vi "HFRR ADV v08.vi"() -> ()   [LabVIEW 2025] (continued)
                        "Humidity 2" <- w4456
                        n3193 = local write "Send"(w4457) -> ()
                        n3194 = local write "Ser Led"(w4457) -> ()
                        n3195 = VISA Read(VISA resource name=w4463, byte count=w4456, error in (no error)=w4464) -> (VISA resource name out=w4460:refnum<visa-resource-name>, read buffer=→"Humidity Str Rec":string, error out=w4459:errorcluster)  [unwired: 1 out]
                      }
                    }
                    n3196 = Select(t=w4434, s=w4435, f=w4432) -> (s? t:f=w4433:string)
                  }
                }
              }
              frame Error {
                w4480 = u16 0 items=["None"=0, "XON/XOFF"=1, "RTS/CTS"=2, "DTR/DSR"=4] ("flow control")
                w4476 = u16 0 items=["None", "Odd", "Even", "Mark", "Space"] ("parity")
                w4479 = u16 10 items=["1.0"=10, "1.5"=15, "2.0"=20] ("stop bits")
                n3197 = VISA Close(VISA resource name=w4472, error in (no error)=w4473) -> (error out=w4471:errorcluster)
                n3198 = local write "humid"("" ("humid")) -> ()
                n3199 = local write "Humidity Str Rec"("" ("Humidity Str Rec")) -> ()
                n3200 = call <vilib>:"Clear Errors.vi"("error in (no error)"=w4471) -> ("error out"=w4470:errorcluster)  [unwired: 5 in, 1 out]
                n3201 = local read "Com Port 3"() -> (w4469:refnum<visa-resource-name>)
                n3202 = call-poly "VISA Configure Serial Port"("VISA resource name"=w4469, "timeout (10sec)"=u32 1000, "termination char\n(0xA = '\\n' = LF)"=u8 10 ("termination char\n(0xA = '\\n' = LF)"), "Enable Termination\nChar (T)"=FALSE ("Enable Termination Char (T)"), "baud rate (9600)"="Humidity BaudRate", "data bits (8)"=u16 8 ("data bits"), "parity (0:none)"=w4476, "error in (no error)"=w4470, "stop bits (10: 1 bit)"=w4479, "flow control (0:none)"=w4480) -> ("VISA resource name out"=w4475:refnum<visa-resource-name>, "error out"=w4466:errorcluster)  [unwired: 4 in]
              }
            }
            n3203 = Compound Arithmetic op=AND(w4371, w4370, w4372) -> (w4369:bool)
            n3204 = case shown="True" w4369 {
              tunnel: w4368 -> [_ _]
              tunnel: w4377 -> [_ w4407]
              frame False {
              }
              frame True {
                w4405 = " " ("regular expression")
                n3205 = Match Pattern(string=w4407, regular expression=" ") -> (after substring=w4409:string)  [unwired: 1 in, 3 out]
                n3206 = Match Pattern(string=w4409, regular expression=w4405) -> (before substring=→"humid":string, after substring=w4406:string)  [unwired: 1 in, 2 out]
                n3207 = Match Pattern(string=w4406, regular expression=w4405) -> (before substring=→"temp_@Rh sensor":string)  [unwired: 1 in, 3 out]
              }
            }
            n3208 = local read "Quit"() -> (w4358:bool)
          }
          n3209 = VISA Close(VISA resource name=w4354, error in (no error)=w4355) -> (error out=w4351:errorcluster)
          n3210 = call <vilib>:"Clear Errors.vi"("error in (no error)"=w4351) -> ()  [unwired: 5 in, 2 out]
        }
        frame Enabled {
        }
      }
    }
    frame Enabled {
    }
  }
  n3211 = while {
    tunnel: [w4488] -> _
    i -> [w4488]
    stop <- w4483 stop-if-true
    # "Langauage selection"
    n3212 = property on="FF Calibration g" class="WFGraph (strict)"("Plot Area:Colors:FG Color"=u32 0) -> ()  [unwired: 2 in, 2 out]
    n3213 = Equal?(x="Lan flag", y=22.0) -> ()  [unwired: 1 out]
    n3214 = disable-structure shown="Disabled" {
      frame Disabled {
        n3215 = stacked-sequence {
          frame #0 {
            n3216 = case shown="\"Russian\"" "Language Selection" {
              tunnel: [0 1] -> w4490
              frame "English", Default {
              }
              frame "Russian" {
              }
            }
            n3217 = for {
              N: 130 -> [_]
              tunnel: "Table" -> [w4499]
              tunnel: w4490 -> [w4498]
              i -> [w4497]
              n3218 = Index Array(array=w4499, index (row)=w4497, index (col)=w4498) -> (element=w4496:string)
              n3219 = case shown="123" w4497 {
                tunnel: w4496 -> [w4500 w4501 _ w4502 w4503 w4504 w4505 w4506 w4507 w4508 w4509 w4510 w4511 w4512 w4513 w4514 w4515 w4516 w4517 w4518 w4519 w4520 w4521 w4522 w4523 w4524 w4525 w4526 w4527 _ _ w4528 w4529 w4530 w4531 w4532 w4533 w4542 w4549 w4556 w4563 w4567 w4570 w4573 w4575 w4577 w4578 w4579 w4580 w4581 w4582 w4583 w4584 w4585 w4586 w4587 w4588 w4589 w4590 w4591 w4592 w4593 w4594 w4595 w4596 w4597 w4598 w4599 w4600 w4601 w4602 w4603 w4604 w4605 w4606 w4607 w4608 w4609 w4610 w4611 w4612 w4613 w4614 w4615 w4616 w4617 w4618 w4619 w4620 w4621 w4622 w4623 w4624 w4625 w4626 w4627 w4628 w4629 w4630 w4631 w4632 w4633 w4634 w4635 w4636 _ w4637 w4638 w4639 w4640 w4641 w4642 w4643 w4644 w4645 w4646 w4647 w4648 w4649 _ w4650 w4651 w4652 w4653 w4654 w4655 _]
                frame 0 {
                  n3220 = local write "S"(w4500) -> ()
                }
                frame 1 {
                  n3221 = local write "S 2"(w4501) -> ()
                }
                frame 2 {
                }
                frame 3 {
                  n3222 = local write "S 4"(w4502) -> ()
                }
                frame 4 {
                  n3223 = property on="FILE" class="Str"("Caption.Text"=w4503) -> ()  [unwired: 2 in, 2 out]
                }
                frame 5 {
                  n3224 = property on="Fuel Discription :" class="Str"("Caption.Text"=w4504) -> ()  [unwired: 2 in, 2 out]
                }
                frame 6 {
                  n3225 = property on="Remarks :" class="Str"("Caption.Text"=w4505) -> ()  [unwired: 2 in, 2 out]
                }
                frame 7 {
                  n3226 = property on="Save & Continue" class="Bool (strict)"("Boolean Text.Text"=w4506) -> ()  [unwired: 2 in, 2 out]
                }
                frame 8 {
                }
                frame 9 {
                  n3227 = property on="Set Hz" class="DigNum (strict)"("Caption.Text"=w4508) -> ()  [unwired: 2 in, 2 out]
                }
                frame 10 {
                  "String 3" <- w4509
                }
                frame 11 {
                  n3228 = property on="NORMAL LOAD" class="DigNum (strict)"("Caption.Text"=w4510) -> ()  [unwired: 2 in, 2 out]
                }
                frame 12 {
                  "String 5" <- w4511
                }
                frame 13 {
                  n3229 = property on="Set Temp" class="DigNum (strict)"("Caption.Text"=w4512) -> ()  [unwired: 2 in, 2 out]
                }
                frame 14 {
                  n3230 = local write "S 15"(w4513) -> ()
                }
                frame 15 {
                  n3231 = property on="Set Rh" class="DigNum (strict)"("Caption.Text"=w4514) -> ()  [unwired: 2 in, 2 out]
                }
                frame 16 {
                  "String 13" <- w4515
                  "String 26" <- w4515
                }
                frame 17 {
                  n3232 = local write "S 18"(w4516) -> ()
                }
                frame 18 {
                  "String 17" <- w4517
                }
                frame 19 {
                  n3233 = property on="test time" class="DigNum (strict)"("Caption.Text"=w4518) -> ()  [unwired: 2 in, 2 out]
                }
                frame 20 {
                  "String 18" <- w4519
                  "String 22" <- w4519
                }
                frame 21 {
                  n3234 = property on="Elapsed time" class="DigNum (strict)"("Caption.Text"=w4520) -> ()  [unwired: 2 in, 2 out]
                }
                frame 22 {
                  n3235 = property on="Samplingtime 2" class="DigNum (strict)"("Caption.Text"=w4521) -> ()  [unwired: 2 in, 2 out]
                }
                frame 23 {
                  "String 21" <- w4522
                }
                frame 24 {
                  n3236 = property on="Countdown" class="DigNum (strict)"("Caption.Text"=w4523) -> ()  [unwired: 2 in, 2 out]
                }
                frame 25 {
                  n3237 = property on="Countdown 2" class="DigNum (strict)"("Caption.Text"=w4524) -> ()  [unwired: 2 in, 2 out]
                }
                frame 26 {
                  n3238 = property on="Engage" class="Bool (strict)"("Boolean Text.Text"=w4525) -> ()  [unwired: 2 in, 2 out]
                }
                frame 27 {
                  n3239 = property on="Boolean  4" class="Bool (strict)"("Boolean Text.Text"=w4526) -> ()  [unwired: 2 in, 2 out]
                }
                frame 28 {
                  n3240 = property on="Test \nStatus" class="Bool (strict)"("Boolean Text.Text"=w4527) -> ()  [unwired: 2 in, 2 out]
                }
                frame 29 {
                }
                frame 30 {
                }
                frame 31 {
                  n3241 = property on="FF Calibration g" class="WFGraph (strict)"("X Scale.Name Label.Text"=w4528) -> ()  [unwired: 2 in, 2 out]
                }
                frame 32 {
                  n3242 = property on="RSTCOF" class="Bool"("Boolean Text.Text"=w4529) -> ()  [unwired: 2 in, 2 out]
                  n3243 = property on="RST FF" class="Bool"("Boolean Text.Text"=w4529) -> ()  [unwired: 2 in, 2 out]
                  n3244 = property on="RST TEMP" class="Bool"("Boolean Text.Text"=w4529) -> ()  [unwired: 2 in, 2 out]
                  n3245 = property on="RSTV1 3" class="Bool"("Boolean Text.Text"=w4529) -> ()  [unwired: 2 in, 2 out]
                  n3246 = property on="rstv2" class="Bool"("Boolean Text.Text"=w4529) -> ()  [unwired: 2 in, 2 out]
                  n3247 = property on="RSTV1 2" class="Bool"("Boolean Text.Text"=w4529) -> ()  [unwired: 2 in, 2 out]
                  n3248 = property on="RST CP" class="Bool"("Boolean Text.Text"=w4529) -> ()  [unwired: 2 in, 2 out]
                }
                frame 33 {
                  "S 61" <- w4530
                }
                frame 34 {
                  "String 23" <- w4531
                }
                frame 35 {
                  n3249 = property on="Rh Before" class="DigNum (strict)"("Caption.Text"=w4532) -> ()  [unwired: 2 in, 2 out]
                }
                frame 36 {
                  n3250 = Match Pattern(string=w4533, regular expression=",") -> (before substring=→"bs":string, after substring=→"as":string)  [unwired: 1 in, 2 out]
                  n3251 = property on="Rh After" class="DigNum (strict)"("Caption.Text"=w4533) -> ()  [unwired: 2 in, 2 out]
                }
                frame 37 {
                  n3252 = Match Pattern(string=w4542, regular expression=",") -> (before substring=w4541:string, after substring=w4540:string)  [unwired: 1 in, 2 out]
                  "bs" <- w4541
                  "as" <- w4540
                  n3253 = Concatenate Strings(w4541, w4540) -> (w4537:string)
                  n3254 = property on="Humidity before test 2" class="DigNum (strict)"("Caption.Text"=w4537) -> ()  [unwired: 2 in, 2 out]
                  n3255 = property on="Humidity before test" class="DigNum (strict)"("Caption.Text"=w4537) -> ()  [unwired: 2 in, 2 out]
                  n3256 = Concatenate Strings(w4537, "=" ("string")) -> (w4538:string)
                  n3257 = local write "S 38"(w4538) -> ()
                }
                frame 38 {
                  n3258 = Match Pattern(string=w4549, regular expression=",") -> (before substring=w4548:string, after substring=w4547:string)  [unwired: 1 in, 2 out]
                  "bs" <- w4548
                  "as" <- w4547
                  n3259 = Concatenate Strings(w4548, w4547) -> (w4544:string)
                  n3260 = property on="Humidity after test 2" class="DigNum (strict)"("Caption.Text"=w4544) -> ()  [unwired: 2 in, 2 out]
                  n3261 = Concatenate Strings(w4544, "=" ("string")) -> (w4546:string)
                  n3262 = property on="Humidity after test" class="DigNum (strict)"("Caption.Text"=w4544) -> ()  [unwired: 2 in, 2 out]
                  n3263 = local write "S 39"(w4546) -> ()
                }
                frame 39 {
                  n3264 = Match Pattern(string=w4556, regular expression=",") -> (before substring=w4555:string, after substring=w4554:string)  [unwired: 1 in, 2 out]
                  "bs" <- w4555
                  "as" <- w4554
                  n3265 = Concatenate Strings(w4555, w4554) -> (w4551:string)
                  n3266 = property on="Temperature before test 2" class="DigNum (strict)"("Caption.Text"=w4551) -> ()  [unwired: 2 in, 2 out]
                  n3267 = property on="Temperature before test" class="DigNum (strict)"("Caption.Text"=w4551) -> ()  [unwired: 2 in, 2 out]
                  n3268 = Concatenate Strings(w4551, "=" ("string")) -> (→"String 34":string)
                }
                frame 40 {
                  n3269 = Match Pattern(string=w4563, regular expression=",") -> (before substring=w4562:string, after substring=w4561:string)  [unwired: 1 in, 2 out]
                  "bs" <- w4562
                  "as" <- w4561
                  n3270 = Concatenate Strings(w4562, w4561) -> (w4558:string)
                  n3271 = property on="Temperature after test 2" class="DigNum (strict)"("Caption.Text"=w4558) -> ()  [unwired: 2 in, 2 out]
                  n3272 = Concatenate Strings(w4558, "=" ("string")) -> (→"String 35":string)
                  n3273 = property on="Temperature after test" class="DigNum (strict)"("Caption.Text"=w4558) -> ()  [unwired: 2 in, 2 out]
                }
                frame 41 {
                  n3274 = property on="AVP" class="DigNum (strict)"("Caption.Text"=w4567) -> ()  [unwired: 2 in, 2 out]
                  n3275 = property on="AVP 2" class="DigNum (strict)"("Caption.Text"=w4567) -> ()  [unwired: 2 in, 2 out]
                  n3276 = Concatenate Strings(w4567, "=" ("string")) -> (→"String 36":string)
                }
                frame 42 {
                  n3277 = property on="MWSD" class="DigNum (strict)"("Caption.Text"=w4570) -> ()  [unwired: 2 in, 2 out]
                  n3278 = property on="MWSD 2" class="DigNum (strict)"("Caption.Text"=w4570) -> ()  [unwired: 2 in, 2 out]
                  n3279 = Concatenate Strings(w4570, "=" ("string")) -> (→"String 37":string)
                }
                frame 43 {
                  n3280 = property on="HCF 2" class="DigNum (strict)"("Caption.Text"=w4573) -> ()  [unwired: 2 in, 2 out]
                  n3281 = property on="HCF" class="DigNum (strict)"("Caption.Text"=w4573) -> ()  [unwired: 2 in, 2 out]
                  n3282 = Concatenate Strings(w4573, "=" ("string")) -> (→"String 38":string)
                }
                frame 44 {
                  n3283 = Concatenate Strings(w4575, "=" ("string")) -> (→"String 39":string)
                  n3284 = property on="WS1.4 2" class="DigNum (strict)"("Caption.Text"=w4575) -> ()  [unwired: 2 in, 2 out]
                  n3285 = property on="WS1.4" class="DigNum (strict)"("Caption.Text"=w4575) -> ()  [unwired: 2 in, 2 out]
                }
                frame 45 {
                  n3286 = property on="Save Results" class="Bool (strict)"("Boolean Text.Text"=w4577) -> ()  [unwired: 2 in, 2 out]
                }
                frame 46 {
                  n3287 = local write "S 47"(w4578) -> ()
                }
                frame 47 {
                  n3288 = local write "S 48"(w4579) -> ()
                }
                frame 48 {
                  n3289 = local write "S 49"(w4580) -> ()
                }
                frame 49 {
                  n3290 = local write "S 50"(w4581) -> ()
                }
                frame 50 {
                  n3291 = local write "S 51"(w4582) -> ()
                }
                frame 51 {
                  n3292 = local write "S 52"(w4583) -> ()
                }
                frame 52 {
                  n3293 = local write "S 53"(w4584) -> ()
                }
                frame 53 {
                  n3294 = local write "S 54"(w4585) -> ()
                }
                frame 54 {
                  n3295 = local write "S 55"(w4586) -> ()
                }
                frame 55 {
                  n3296 = local write "S 56"(w4587) -> ()
                }
                frame 56 {
                  n3297 = local write "S 57"(w4588) -> ()
                }
                frame 57 {
                  n3298 = local write "S 58"(w4589) -> ()
                }
                frame 58 {
                  n3299 = local write "S 59"(w4590) -> ()
                }
                frame 59 {
                  n3300 = local write "S 60"(w4591) -> ()
                }
                frame 60 {
                  n3301 = local write "S 62"(w4592) -> ()
                }
                frame 61 {
                  n3302 = local write "S 63"(w4593) -> ()
                }
                frame 62 {
                  n3303 = local write "S 64"(w4594) -> ()
                }
                frame 63 {
                  n3304 = local write "S 65"(w4595) -> ()
                }
                frame 64 {
                  n3305 = local write "S 66"(w4596) -> ()
                }
                frame 65 {
                  n3306 = local write "S 67"(w4597) -> ()
                }
                frame 66 {
                  n3307 = local write "S 68"(w4598) -> ()
                }
                frame 67 {
                  n3308 = local write "S 69"(w4599) -> ()
                }
                frame 68 {
                  n3309 = local write "S 70"(w4600) -> ()
                }
                frame 69 {
                  n3310 = local write "S 71"(w4601) -> ()
                }
                frame 70 {
                  n3311 = local write "S 72"(w4602) -> ()
                }
                frame 71 {
                  n3312 = local write "S 73"(w4603) -> ()
                }
                frame 72 {
                  n3313 = local write "S 74"(w4604) -> ()
                }
                frame 73 {
                  n3314 = local write "S 75"(w4605) -> ()
                }
                frame 74 {
                  n3315 = local write "S 76"(w4606) -> ()
                }
                frame 75 {
                  n3316 = local write "S 77"(w4607) -> ()
                }
                frame 76 {
                  n3317 = local write "S 78"(w4608) -> ()
                }
                frame 77 {
                  n3318 = local write "S 79"(w4609) -> ()
                }
                frame 79 {
                  n3319 = property on="Sample Temperature ( °C )" class="XYGraph (strict)"("Y Scale.Name Label.Text"=w4610) -> ()  [unwired: 2 in, 2 out]
                }
                frame 80 {
                  n3320 = local write "S 81"(w4611) -> ()
                  n3321 = property on="Humidity ( %RH )" class="XYGraph (strict)"("Y Scale.Name Label.Text"=w4611) -> ()  [unwired: 2 in, 2 out]
                }
                frame 78 {
                  n3322 = property on="Air Temperature  ( °C )" class="XYGraph (strict)"("X Scale.Name Label.Text"=w4612) -> ()  [unwired: 2 in, 2 out]
                  n3323 = property on="Humidity ( %RH )" class="XYGraph (strict)"("X Scale.Name Label.Text"=w4612) -> ()  [unwired: 2 in, 2 out]
                  n3324 = property on="Sample Temperature ( °C )" class="XYGraph (strict)"("X Scale.Name Label.Text"=w4612) -> ()  [unwired: 2 in, 2 out]
                  n3325 = property on="Coefficient Of Friction" class="XYGraph (strict)"("X Scale.Name Label.Text"=w4612) -> ()  [unwired: 2 in, 2 out]
                }
                frame 81 {
                  n3326 = property on="Air Temperature  ( °C )" class="XYGraph (strict)"("Y Scale.Name Label.Text"=w4613) -> ()  [unwired: 2 in, 2 out]
                }
                frame 82 {
                  n3327 = local write "S 84"(w4614) -> ()
                }
                frame 83 {
                  n3328 = local write "S 85"(w4615) -> ()
                }
                frame 84 {
                  n3329 = local write "S 86"(w4616) -> ()
                }
                frame 85 {
                  n3330 = local write "S 87"(w4617) -> ()
                }
                frame 86 {
                  n3331 = local write "S 88"(w4618) -> ()
                }
                frame 87 {
                  n3332 = property on="FF Calibration g" class="WFGraph (strict)"("Y Scale.Name Label.Text"=w4619) -> ()  [unwired: 2 in, 2 out]
                }
                frame 88 {
                  n3333 = local write "S 90"(w4620) -> ()
                }
                frame 89 {
                  n3334 = local write "S 91"(w4621) -> ()
                }
                frame 90 {
                  n3335 = local write "S 92"(w4622) -> ()
                }
                frame 91 {
                  n3336 = local write "S 93"(w4623) -> ()
                }
                frame 92 {
                  n3337 = local write "S 94"(w4624) -> ()
                }
                frame 93 {
                  n3338 = local write "S 95"(w4625) -> ()
                }
                frame 94 {
                  n3339 = local write "S 96"(w4626) -> ()
                }
                frame 95 {
                  n3340 = local write "S 97"(w4627) -> ()
                }
                frame 96 {
                  n3341 = local write "S 98"(w4628) -> ()
                }
                frame 97 {
                  n3342 = local write "S 99"(w4629) -> ()
                }
                frame 98 {
                  n3343 = local write "S 100"(w4630) -> ()
                }
                frame 99 {
                  n3344 = local write "S 101"(w4631) -> ()
                }
                frame 100 {
                  n3345 = local write "S 102"(w4632) -> ()
                }
                frame 101 {
                  n3346 = local write "S 103"(w4633) -> ()
                }
                frame 102 {
                  n3347 = local write "S 104"(w4634) -> ()
                }
                frame 103 {
                  n3348 = local write "S 105"(w4635) -> ()
                }
                frame 104 {
                  n3349 = local write "S 106"(w4636) -> ()
                }
                frame 105 {
                }
                frame 106 {
                  n3350 = property on="OK Button 17" class="Bool (strict)"("Boolean Text.Text"=w4637) -> ()  [unwired: 2 in, 2 out]
                }
                frame 107 {
                  n3351 = property on="OK Button 16" class="Bool (strict)"("Boolean Text.Text"=w4638) -> ()  [unwired: 2 in, 2 out]
                }
                frame 108 {
                  n3352 = property on="TITTLE" class="Str"("Caption.Text"=w4639) -> ()  [unwired: 2 in, 2 out]
                }
                frame 109 {
                  "String 30" <- w4640
                }
                frame 110 {
                  n3353 = property on="Test Date" class="Str"("Caption.Text"=w4641) -> ()  [unwired: 2 in, 2 out]
                  "String 31" <- w4641
                }
                frame 111 {
                  n3354 = property on="Sample ID" class="Str"("Caption.Text"=w4642) -> ()  [unwired: 2 in, 2 out]
                  "String 32" <- w4642
                }
                frame 112 {
                  n3355 = property on="Tested by" class="Str"("Caption.Text"=w4643) -> ()  [unwired: 2 in, 2 out]
                  "String 33" <- w4643
                }
                frame 113 {
                  n3356 = property on="System Configured Printers 2" class="Arr (strict)"("Caption.Text"=w4644) -> ()  [unwired: 2 in, 2 out]
                }
                frame 114 {
                  n3357 = property on="Selected Printer" class="Str"("Caption.Text"=w4645) -> ()  [unwired: 2 in, 2 out]
                }
                frame 115 {
                  n3358 = property on="Select Printer 3" class="DigNum (strict)"("Caption.Text"=w4646) -> ()  [unwired: 2 in, 2 out]
                }
                frame 116 {
                  n3359 = property on="Print" class="Bool (strict)"("Boolean Text.Text"=w4647) -> ()  [unwired: 2 in, 2 out]
                }
                frame 117 {
                  "String 41" <- w4648
                }
                frame 118 {
                  n3360 = property on="tested by" class="Str"("Caption.Text"=w4649) -> ()  [unwired: 2 in, 2 out]
                }
                frame 119 {
                }
                frame 120 {
                  n3361 = property on="Export" class="Bool (strict)"("Boolean Text.Text"=w4650) -> ()  [unwired: 2 in, 2 out]
                }
                frame 121 {
                  n3362 = property on="TEMP INTERCEPT:" class="DigNum (strict)"("Caption.Text"=w4651) -> ()  [unwired: 2 in, 2 out]
                }
                frame 122 {
                  n3363 = property on="AIR TEMP INTERCEPT:" class="DigNum (strict)"("Caption.Text"=w4652) -> ()  [unwired: 2 in, 2 out]
                }
                frame 123 {
                  n3364 = property on="Select File Type" class="Enum (strict)"("Caption.Text"=w4653) -> ()  [unwired: 2 in, 2 out]
                }
                frame 124 {
                  n3365 = property on="s.NO" class="Str"("Caption.Text"=w4654) -> ()  [unwired: 2 in, 2 out]
                  "String 45" <- w4654
                }
                frame 125 {
                  n3366 = property on="trip1 8" class="Bool (strict)"("Boolean Text.Text"=w4655) -> ()  [unwired: 2 in, 2 out]
                }
                frame 126, Default {
                }
              }
            }
          }
          frame #1 {
            w4663 = TRUE ("Visible")
            n3367 = local read "S 91"() -> (w4680:string)
            n3368 = local read "S 90"() -> (w4679:string)
            n3369 = local read "S 88"() -> (w4678:string)
            n3370 = property on="Threshold" class="DigNum (strict)"("Caption.Text"=w4680) -> ()  [unwired: 2 in, 2 out]
            n3371 = property on="File Path" class="Path"("Caption.Text"=w4679) -> ()  [unwired: 2 in, 2 out]
            n3372 = property on="SrvM CP" class="Bool (strict)"("Boolean Text.Text"=w4678) -> ()  [unwired: 2 in, 2 out]
            n3373 = local read "S 71"() -> (w4673:string)
            n3374 = local read "S 86"() -> (w4675:string)
            n3375 = local read "S 85"() -> (w4676:string)
            n3376 = local read "S 87"() -> (w4674:string)
            n3377 = local read "S 84"() -> (w4677:string)
            n3378 = local read "S 103"() -> (w4662:string)
            n3379 = local read "S 104"() -> (w4661:string)
            n3380 = property on="ENTER THE NEW PASSWORD" class="Str"("Caption.Text"=w4674) -> ()  [unwired: 2 in, 2 out]
            n3381 = property on="Password" class="Str"("Caption.Text"=w4676) -> ()  [unwired: 2 in, 2 out]
            n3382 = property on="ENTER CURRENT PASSWORD" class="Str"("Caption.Text"=w4675) -> ()  [unwired: 2 in, 2 out]
            n3383 = property on="EDIT" class="Bool (strict)"("Boolean Text.Text"=w4673) -> ()  [unwired: 2 in, 2 out]
            n3384 = property on="SAVE" class="Bool (strict)"("Boolean Text.Text"=w4677) -> ()  [unwired: 2 in, 2 out]
            n3385 = Build Array(w4662, w4661) -> (w4660:string[])
            n3386 = property on="Heater Button" class="Bool (strict)"("Strings [4]"=w4660) -> ()  [unwired: 2 in, 2 out]
            n3387 = property on="CH-HUMIDITY WET" class="DigNum (strict)"("Caption.Size to Text?"=w4663) -> ()  [unwired: 2 in, 2 out]
            n3388 = property on="CH-HUMIDITY DRY" class="DigNum (strict)"("Caption.Size to Text?"=w4663) -> ()  [unwired: 2 in, 2 out]
            n3389 = property on="CH-POWER -" class="DigNum (strict)"("Caption.Size to Text?"=w4663) -> ()  [unwired: 2 in, 2 out]
            n3390 = property on="CH-HEATER" class="DigNum (strict)"("Caption.Size to Text?"=w4663) -> ()  [unwired: 2 in, 2 out]
            n3391 = property on="CH-POWER +" class="DigNum (strict)"("Caption.Size to Text?"=w4663) -> ()  [unwired: 2 in, 2 out]
            n3392 = local read "S 92"() -> (w4672:string)
            n3393 = local read "S 93"() -> (w4671:string)
            n3394 = local read "S 105"() -> (w4658:string)
            n3395 = local read "S 106"() -> (w4657:string)
            n3396 = Build Array(w4672, w4671) -> ()  [unwired: 1 out]
            n3397 = Build Array(w4658, w4657) -> (w4659:string[])
            n3398 = local read "S 95"() -> (w4669:string)
            n3399 = local read "S 94"() -> (w4670:string)
            n3400 = local read "bs"() -> (w4685:string)
            n3401 = local read "as"() -> (w4686:string)
            n3402 = property on="Humidity" class="Bool (strict)"("Strings [4]"=w4659) -> ()  [unwired: 2 in, 2 out]
            n3403 = Concatenate Strings(w4685, "\r", w4686) -> ()  [unwired: 1 out]
            n3404 = property on="STROKE GAIN :" class="DigNum (strict)"("Caption.Text"=w4669) -> ()  [unwired: 2 in, 2 out]
            n3405 = property on="DISPLACEMENT :" class="DigNum (strict)"("Caption.Text"=w4670) -> ()  [unwired: 2 in, 2 out]
            n3406 = property on="Rh After" class="DigNum (strict)"("Caption.Size to Text?"=TRUE ("Caption.Size to Text")) -> ()  [unwired: 2 in, 2 out]
            n3407 = local read "S 48"() -> (w4709:string)
            n3408 = local read "S 50"() -> (w4707:string)
            n3409 = local read "S 51"() -> (w4706:string)
            n3410 = local read "S 49"() -> (w4708:string)
            n3411 = local read "S 52"() -> (w4705:string)
            n3412 = local read "as"() -> (w4690:string)
            n3413 = local read "bs"() -> (w4691:string)
            n3414 = local read "S 56"() -> (w4704:string)
            n3415 = local read "S 57"() -> (w4703:string)
            n3416 = local read "S 58"() -> (w4702:string)
            n3417 = local read "S 59"() -> (w4701:string)
            n3418 = property on="OPEN" class="Bool (strict)"("Boolean Text.Text"=w4705) -> ()  [unwired: 2 in, 2 out]
            n3419 = property on="OPEN 1" class="Bool (strict)"("Boolean Text.Text"=w4709) -> ()  [unwired: 2 in, 2 out]
            n3420 = property on="OPEN 2" class="Bool (strict)"("Boolean Text.Text"=w4708) -> ()  [unwired: 2 in, 2 out]
            n3421 = property on="OPEN 3" class="Bool (strict)"("Boolean Text.Text"=w4707) -> ()  [unwired: 2 in, 2 out]
            n3422 = property on="OPEN 4" class="Bool (strict)"("Boolean Text.Text"=w4706) -> ()  [unwired: 2 in, 2 out]
            n3423 = Concatenate Strings(w4691, "\r", w4690) -> ()  [unwired: 1 out]
            n3424 = local read "S 102"() -> (w4664:string)
            n3425 = property on="КОФ1" class="DigNum (strict)"("Caption.Text"=w4704) -> ()  [unwired: 2 in, 2 out]
            n3426 = local read "S 98"() -> (w4668:string)
            n3427 = local read "S 99"() -> (w4667:string)
            n3428 = local read "S 100"() -> (w4666:string)
            n3429 = local read "S 101"() -> (w4665:string)
            n3430 = property on="КОФ2" class="DigNum (strict)"("Caption.Text"=w4703) -> ()  [unwired: 2 in, 2 out]
            n3431 = property on="КОФ3" class="DigNum (strict)"("Caption.Text"=w4702) -> ()  [unwired: 2 in, 2 out]
            n3432 = property on="КОФ4" class="DigNum (strict)"("Caption.Text"=w4701) -> ()  [unwired: 2 in, 2 out]
            n3433 = local read "bs"() -> (w4689:string)
            n3434 = local read "as"() -> (w4688:string)
            n3435 = property on="CH-POWER +" class="DigNum (strict)"("Caption.Text"=w4668) -> ()  [unwired: 2 in, 2 out]
            n3436 = property on="CH-POWER -" class="DigNum (strict)"("Caption.Text"=w4667) -> ()  [unwired: 2 in, 2 out]
            n3437 = property on="CH-HEATER" class="DigNum (strict)"("Caption.Text"=w4666) -> ()  [unwired: 2 in, 2 out]
            n3438 = property on="CH-HUMIDITY DRY" class="DigNum (strict)"("Caption.Text"=w4665) -> ()  [unwired: 2 in, 2 out]
            n3439 = property on="CH-HUMIDITY WET" class="DigNum (strict)"("Caption.Text"=w4664) -> ()  [unwired: 2 in, 2 out]
            n3440 = local read "S 60"() -> (w4700:string)
            n3441 = local read "S 54"() -> (w4710:string)
            n3442 = Concatenate Strings(w4689, "\r", w4688) -> ()  [unwired: 1 out]
            n3443 = Concatenate Strings(w4710, w4700) -> ()  [unwired: 1 out]
            n3444 = local read "S 77"() -> (→"String 43":string)
            n3445 = local read "S 76"() -> (w4683:string)
            n3446 = local read "S 78"() -> (w4682:string)
            n3447 = local read "S 71"() -> (w4694:string)
            n3448 = local read "S 66"() -> (w4699:string)
            n3449 = local read "S 67"() -> (w4698:string)
            n3450 = local read "S 68"() -> (w4697:string)
            n3451 = local read "S 69"() -> (w4696:string)
            n3452 = local read "S 70"() -> (w4695:string)
            n3453 = property on="AIR TEMP" class="DigNum (strict)"("Caption.Text"=w4682) -> ()  [unwired: 2 in, 2 out]
            n3454 = property on="Set Strk" class="DigNum (strict)"("Caption.Text"=w4683) -> ()  [unwired: 2 in, 2 out]
            n3455 = property on="FRIC. FORCE :" class="DigNum (strict)"("Caption.Text"=w4699) -> ()  [unwired: 2 in, 2 out]
            n3456 = property on="TEMPERATURE :" class="DigNum (strict)"("Caption.Text"=w4698) -> ()  [unwired: 2 in, 2 out]
            n3457 = property on="SPEED OUT:" class="DigNum (strict)"("Caption.Text"=w4697) -> ()  [unwired: 2 in, 2 out]
            n3458 = property on="AIR TEMPERATURE :" class="DigNum (strict)"("Caption.Text"=w4696) -> ()  [unwired: 2 in, 2 out]
            n3459 = property on="HUMIDITY:" class="DigNum (strict)"("Caption.Text"=w4695) -> ()  [unwired: 2 in, 2 out]
            n3460 = property on="EDIT" class="Bool (strict)"("Boolean Text.Text"=w4694) -> ()  [unwired: 2 in, 2 out]
            n3461 = local read "S 79"() -> (w4681:string)
            n3462 = property on="Stroke" class="DigNum (strict)"("Caption.Text"=w4681) -> ()  [unwired: 2 in, 2 out]
          }
          frame #2 {
          }
        }
        n3463 = local write "Lan flag"(10.0 ("Lan flag")) -> ()
      }
      frame Enabled {
      }
    }
    n3464 = Wait (ms)(milliseconds to wait=u32 2000) -> ()  [unwired: 1 out]
    n3465 = local read "Quit"() -> (w4483:bool)
  }
  n3466 = disable-structure shown="Disabled" {
    frame Disabled {
      n3467 = while {
        tunnel: [w4712] -> _
        i -> [w4712]
        stop <- w4711 continue-if-true
        n3468 = Wait (ms)(milliseconds to wait=u32 50) -> ()  [unwired: 1 out]
        n3469 = stacked-sequence {
          frame #0 {
            # "Controls Text color"
            # "Controls BG color"
            n3470 = property on="FILE" class="Str"("Text.Text Colors:Text Color"="SC  Text") -> ()  [unwired: 2 in, 2 out]
            n3471 = property on="Fuel Discription :" class="Str"("Text.Text Colors:Text Color"="SC  Text") -> ()  [unwired: 2 in, 2 out]
            n3472 = property on="tested by" class="Str"("Text.Text Colors:Text Color"="SC  Text") -> ()  [unwired: 2 in, 2 out]
            n3473 = property on="Remarks :" class="Str"("Text.Text Colors:Text Color"="SC  Text") -> ()  [unwired: 2 in, 2 out]
            n3474 = property class="DigNum (strict)"("Numeric Text.Text Colors:BG Color"="NC BG") -> ()  [unwired: 2 in, 2 out]
            n3475 = property class="DigNum (strict)"("Numeric Text.Text Colors:BG Color"="NC BG") -> ()  [unwired: 2 in, 2 out]
            n3476 = property class="DigNum (strict)"("Numeric Text.Text Colors:BG Color"="NC BG") -> ()  [unwired: 2 in, 2 out]
            n3477 = property class="DigNum (strict)"("Numeric Text.Text Colors:BG Color"="NC BG") -> ()  [unwired: 2 in, 2 out]
            n3478 = property class="DigNum (strict)"("Numeric Text.Text Colors:BG Color"="NC BG") -> ()  [unwired: 2 in, 2 out]
            n3479 = property class="DigNum (strict)"("Numeric Text.Text Colors:BG Color"="NC BG") -> ()  [unwired: 2 in, 2 out]
            n3480 = property class="DigNum (strict)"("Numeric Text.Text Colors:BG Color"="NC BG") -> ()  [unwired: 2 in, 2 out]
            n3481 = property class="DigNum (strict)"("Numeric Text.Text Colors:BG Color"="NC BG") -> ()  [unwired: 2 in, 2 out]
            n3482 = property class="DigNum (strict)"("Numeric Text.Text Colors:BG Color"="NC BG") -> ()  [unwired: 2 in, 2 out]
            n3483 = property class="DigNum (strict)"("Numeric Text.Text Colors:BG Color"="NC BG") -> ()  [unwired: 2 in, 2 out]
            n3484 = property class="DigNum (strict)"("Numeric Text.Text Colors:BG Color"="NC BG") -> ()  [unwired: 2 in, 2 out]
            n3485 = property class="DigNum (strict)"("Numeric Text.Text Colors:BG Color"="NC BG") -> ()  [unwired: 2 in, 2 out]
            n3486 = property on="FILE" class="Str"("Text.Text Colors:BG Color"="SC BG 3") -> ()  [unwired: 2 in, 2 out]
            n3487 = property on="Fuel Discription :" class="Str"("Text.Text Colors:BG Color"="SC BG 3") -> ()  [unwired: 2 in, 2 out]
            n3488 = property on="tested by" class="Str"("Text.Text Colors:BG Color"="SC BG 3") -> ()  [unwired: 2 in, 2 out]
            n3489 = property on="Remarks :" class="Str"("Text.Text Colors:BG Color"="SC BG 3") -> ()  [unwired: 2 in, 2 out]
            n3490 = property class="DigNum (strict)"("Numeric Text.Text Colors:Text Color"="NC Text") -> ()  [unwired: 2 in, 2 out]
            n3491 = property class="DigNum (strict)"("Numeric Text.Text Colors:Text Color"="NC Text") -> ()  [unwired: 2 in, 2 out]
            n3492 = property class="DigNum (strict)"("Numeric Text.Text Colors:Text Color"="NC Text") -> ()  [unwired: 2 in, 2 out]
            n3493 = property class="DigNum (strict)"("Numeric Text.Text Colors:Text Color"="NC Text") -> ()  [unwired: 2 in, 2 out]
            n3494 = property class="DigNum (strict)"("Numeric Text.Text Colors:Text Color"="NC Text") -> ()  [unwired: 2 in, 2 out]
            n3495 = property class="DigNum (strict)"("Numeric Text.Text Colors:Text Color"="NC Text") -> ()  [unwired: 2 in, 2 out]
            n3496 = property class="DigNum (strict)"("Numeric Text.Text Colors:Text Color"="NC Text") -> ()  [unwired: 2 in, 2 out]
            n3497 = property class="DigNum (strict)"("Numeric Text.Text Colors:Text Color"="NC Text") -> ()  [unwired: 2 in, 2 out]
            n3498 = property class="DigNum (strict)"("Numeric Text.Text Colors:Text Color"="NC Text") -> ()  [unwired: 2 in, 2 out]
            n3499 = property class="DigNum (strict)"("Numeric Text.Text Colors:Text Color"="NC Text") -> ()  [unwired: 2 in, 2 out]
            n3500 = property class="DigNum (strict)"("Numeric Text.Text Colors:Text Color"="NC Text") -> ()  [unwired: 2 in, 2 out]
            n3501 = property class="DigNum (strict)"("Numeric Text.Text Colors:Text Color"="NC Text") -> ()  [unwired: 2 in, 2 out]
            n3502 = property class="DigNum (strict)"("Numeric Text.Text Colors:Text Color"="NI Text  2") -> ()  [unwired: 2 in, 2 out]
            n3503 = property class="DigNum (strict)"("Numeric Text.Text Colors:Text Color"="NI Text  2") -> ()  [unwired: 2 in, 2 out]
            n3504 = property class="DigNum (strict)"("Numeric Text.Text Colors:Text Color"="NI Text  2") -> ()  [unwired: 2 in, 2 out]
            n3505 = property class="DigNum (strict)"("Numeric Text.Text Colors:Text Color"="NI Text  2") -> ()  [unwired: 2 in, 2 out]
            n3506 = property class="DigNum (strict)"("Numeric Text.Text Colors:Text Color"="NI Text  2") -> ()  [unwired: 2 in, 2 out]
            n3507 = property class="DigNum (strict)"("Numeric Text.Text Colors:Text Color"="NI Text  2") -> ()  [unwired: 2 in, 2 out]
            n3508 = property class="DigNum (strict)"("Numeric Text.Text Colors:Text Color"="NI Text  2") -> ()  [unwired: 2 in, 2 out]
            n3509 = property class="DigNum (strict)"("Numeric Text.Text Colors:Text Color"="NI Text  2") -> ()  [unwired: 2 in, 2 out]
            n3510 = property class="DigNum (strict)"("Numeric Text.Text Colors:Text Color"="NI Text  2") -> ()  [unwired: 2 in, 2 out]
            n3511 = property class="DigNum (strict)"("Numeric Text.Text Colors:Text Color"="NI Text  2") -> ()  [unwired: 2 in, 2 out]
            n3512 = property class="DigNum (strict)"("Numeric Text.Text Colors:Text Color"="NI Text  2") -> ()  [unwired: 2 in, 2 out]
            n3513 = property class="DigNum (strict)"("Numeric Text.Text Colors:Text Color"="NI Text  2") -> ()  [unwired: 2 in, 2 out]
            n3514 = property class="DigNum (strict)"("Numeric Text.Text Colors:Text Color"="NI Text  2") -> ()  [unwired: 2 in, 2 out]
            n3515 = property class="DigNum (strict)"("Numeric Text.Text Colors:Text Color"="NI Text  2") -> ()  [unwired: 2 in, 2 out]
            n3516 = property class="DigNum (strict)"("Numeric Text.Text Colors:Text Color"="NI Text  2") -> ()  [unwired: 2 in, 2 out]
            n3517 = property class="DigNum (strict)"("Numeric Text.Text Colors:Text Color"="NI Text  2") -> ()  [unwired: 2 in, 2 out]
            n3518 = property on="Coefficient Of Friction" class="XYGraph (strict)"("Plot Area:Colors:FG Color"="GFG  2", "Plot Area:Colors:BG Color"="GBG   2") -> ()  [unwired: 2 in, 2 out]
            n3519 = property on="Humidity ( %RH )" class="XYGraph (strict)"("Plot Area:Colors:FG Color"="GFG  2", "Plot Area:Colors:BG Color"="GBG   2") -> ()  [unwired: 2 in, 2 out]
            n3520 = property on="Air Temperature  ( °C )" class="XYGraph (strict)"("Plot Area:Colors:FG Color"="GFG  2", "Plot Area:Colors:BG Color"="GBG   2") -> ()  [unwired: 2 in, 2 out]
            n3521 = property on="Sample Temperature ( °C )" class="XYGraph (strict)"("Plot Area:Colors:FG Color"="GFG  2", "Plot Area:Colors:BG Color"="GBG   2") -> ()  [unwired: 2 in, 2 out]
            n3522 = property class="DigNum (strict)"("Numeric Text.Text Colors:BG Color"="NI BG 2") -> ()  [unwired: 2 in, 2 out]
            n3523 = property class="DigNum (strict)"("Numeric Text.Text Colors:BG Color"="NI BG 2") -> ()  [unwired: 2 in, 2 out]
            n3524 = property class="DigNum (strict)"("Numeric Text.Text Colors:BG Color"="NI BG 2") -> ()  [unwired: 2 in, 2 out]
            n3525 = property class="DigNum (strict)"("Numeric Text.Text Colors:BG Color"="NI BG 2") -> ()  [unwired: 2 in, 2 out]
            n3526 = property class="DigNum (strict)"("Numeric Text.Text Colors:BG Color"="NI BG 2") -> ()  [unwired: 2 in, 2 out]
            n3527 = property class="DigNum (strict)"("Numeric Text.Text Colors:BG Color"="NI BG 2") -> ()  [unwired: 2 in, 2 out]
            n3528 = property class="DigNum (strict)"("Numeric Text.Text Colors:BG Color"="NI BG 2") -> ()  [unwired: 2 in, 2 out]
            n3529 = property class="DigNum (strict)"("Numeric Text.Text Colors:BG Color"="NI BG 2") -> ()  [unwired: 2 in, 2 out]
            n3530 = property class="DigNum (strict)"("Numeric Text.Text Colors:BG Color"="NI BG 2") -> ()  [unwired: 2 in, 2 out]
            n3531 = property class="DigNum (strict)"("Numeric Text.Text Colors:BG Color"="NI BG 2") -> ()  [unwired: 2 in, 2 out]
            n3532 = property class="DigNum (strict)"("Numeric Text.Text Colors:BG Color"="NI BG 2") -> ()  [unwired: 2 in, 2 out]
            n3533 = property class="DigNum (strict)"("Numeric Text.Text Colors:BG Color"="NI BG 2") -> ()  [unwired: 2 in, 2 out]
            n3534 = property class="DigNum (strict)"("Numeric Text.Text Colors:BG Color"="NI BG 2") -> ()  [unwired: 2 in, 2 out]
            n3535 = property class="DigNum (strict)"("Numeric Text.Text Colors:BG Color"="NI BG 2") -> ()  [unwired: 2 in, 2 out]
            n3536 = property class="DigNum (strict)"("Numeric Text.Text Colors:BG Color"="NI BG 2") -> ()  [unwired: 2 in, 2 out]
            n3537 = property class="DigNum (strict)"("Numeric Text.Text Colors:BG Color"="NI BG 2") -> ()  [unwired: 2 in, 2 out]
            n3538 = property class="Bool"("Colors [4]"="Boolean BC T & BG") -> ()  [unwired: 2 in, 2 out]
            n3539 = property on="Save & Continue" class="Bool (strict)"("Colors [4]"="Boolean BC T & BG") -> ()  [unwired: 2 in, 2 out]
            n3540 = property on="Heater Button" class="Bool (strict)"("Colors [4]"="Boolean BC T & BG") -> ()  [unwired: 2 in, 2 out]
            n3541 = property class="Bool"("Colors [4]"="Boolean BC T & BG") -> ()  [unwired: 2 in, 2 out]
            n3542 = property on="Humidity" class="Bool (strict)"("Colors [4]"="Boolean BC T & BG") -> ()  [unwired: 2 in, 2 out]
            n3543 = property class="Bool (strict)"("Colors [4]"="Boolean BC T & BG") -> ()  [unwired: 2 in, 2 out]
            n3544 = property on="RUN" class="Bool (strict)"("Colors [4]"="Boolean BC T & BG") -> ()  [unwired: 2 in, 2 out]
            n3545 = property on="trip1 8" class="Bool (strict)"("Colors [4]"="Boolean BC T & BG") -> ()  [unwired: 2 in, 2 out]
            n3546 = property class="Bool"("Colors [4]"="Boolean BC T & BG") -> ()  [unwired: 2 in, 2 out]
            n3547 = property class="Bool (strict)"("Colors [4]"="Boolean BC T & BG") -> ()  [unwired: 2 in, 2 out]
            n3548 = property on="OPEN 1" class="Bool (strict)"("Colors [4]"="Boolean BC T & BG 2") -> ()  [unwired: 2 in, 2 out]
            n3549 = property on="OPEN 2" class="Bool (strict)"("Colors [4]"="Boolean BC T & BG 2") -> ()  [unwired: 2 in, 2 out]
            n3550 = property on="OPEN 3" class="Bool (strict)"("Colors [4]"="Boolean BC T & BG 2") -> ()  [unwired: 2 in, 2 out]
            n3551 = property on="OPEN 4" class="Bool (strict)"("Colors [4]"="Boolean BC T & BG 2") -> ()  [unwired: 2 in, 2 out]
            n3552 = property on="OPEN" class="Bool (strict)"("Colors [4]"="Boolean BC T & BG 2") -> ()  [unwired: 2 in, 2 out]
            n3553 = property on="rstv2" class="Bool"("Colors [4]"="Boolean BC T & BG 2") -> ()  [unwired: 2 in, 2 out]
            n3554 = property on="RST CP" class="Bool"("Colors [4]"="Boolean BC T & BG 2") -> ()  [unwired: 2 in, 2 out]
            n3555 = property on="RSTV1 3" class="Bool"("Colors [4]"="Boolean BC T & BG 2") -> ()  [unwired: 2 in, 2 out]
            n3556 = property on="RSTV1 2" class="Bool"("Colors [4]"="Boolean BC T & BG 2") -> ()  [unwired: 2 in, 2 out]
          }
          frame #1 {
          }
        }
        n3557 = local read "Quit"() -> (w4711:bool)
      }
    }
    frame Enabled {
    }
  }
  n3558 = while {
    shift-right: [w4729] -> _
    shift-left: _ -> [w4730]
    shift-right: [w4727] -> _
    shift-left: T14 {"Read Heave and Surge"="", "Bytes at Heave Port"=0.0, "Heave and Surge COM Port:"="COM9", "Com Port 2"="COM7", "Residual Due"="", "Heave COM Status 2"=TRUE, "Heave COM Status"=TRUE, "Port 2"=TRUE, "Sway PPR"=6400.0, "Surge PPR"=6400.0, "Heave PPR"=6400.0, "Sway Pitch"=2.0, "Surge Pitch"=3.0, "Heave Pitch"=4.0, "Sway Pulses/mm"=320.0, "Surge Pulses/mm"=1600.0, "Heave Pulses/mm"=1600.0, "inner loop"=0.0, "Read Heave and Surge 2"="", "String 36"="", "Write S"=FALSE, "WriteCC1"=[""], "Heave COM Loop"=0, "LastCom"="", "EXIT"=FALSE, "Error Heave"={"status"=TRUE, "code"=-1073807343, "source"=""}} -> [w4726]
    shift-right: [w4724] -> _
    shift-left: enum16{"init", "MAIN", "Panel Close"}."init" -> [w4725]
    stop <- w4728 stop-if-true
    n3559 = case shown="\"MAIN\"" w4725 {
      tunnel: w4730 -> [w4744 w4759 w4829 w4831]
      tunnel: [w4738 w4777 w4829 w4831] -> w4729
      tunnel: [_ _ TRUE _] -> w4728
      tunnel: [w4734 w4774 w4827 w4830] -> w4727
      tunnel: w4726 -> [w4741 w4758 w4827 w4830]
      tunnel: [enum16{"init", "MAIN", "Panel Close"}."MAIN" w4752 _ _] -> w4724
      frame "init" {
        n3560 = Bundle By Name(cluster=w4741, "Heave and Surge COM Port:"="Humidity :") -> (w4740:T14)
        n3561 = call "Instrument fgv.vi"("Enum"=T23."INIT", "error in (no error) 2"=w4744, "INPUT"=w4740) -> ("error"=w4742:errorcluster, "output"=w4737:T14)  [unwired: 6 in, 1 out]
        n3562 = case shown="No Error" w4742 {
          selector: w4742 -> [w4746 _]
          tunnel: [w4746 w4750] -> w4738
          tunnel: w4737 -> [w4745 w4748]
          tunnel: [w4745 w4747] -> w4735
          frame No Error {
          }
          frame Error {
            n3563 = call "Instrument fgv.vi"("Enum"=T23."ERROR INIT", "INPUT"=w4748) -> ("error"=w4751:errorcluster, "output"=w4747:T14)  [unwired: 7 in, 1 out]
            n3564 = call <vilib>:"Clear Errors.vi"("error in (no error)"=w4751) -> ("error out"=w4750:errorcluster)  [unwired: 5 in, 1 out]
          }
        }
        n3565 = local read "LastCom"() -> (w4733:string)
        n3566 = Unbundle By Name(w4735) -> ("Heave COM Status 2"=→"Heave COM Status 2" →"Instrument Status":bool, "Error Heave"=→"Error Heave":errorcluster)  [unwired: 1 out]
        n3567 = Bundle By Name(cluster=w4735, "LastCom"=w4733) -> (w4734:T14)
      }
      frame "MAIN" {
        n3568 = Unbundle By Name(w4758) -> ("Com Port 2"=w4779:refnum<visa-resource-name>)
        n3569 = local write "Com Port 4"(w4779) -> ()
        n3570 = local read "Humidity :"() -> (w4756:refnum<visa-resource-name>)
        n3571 = Divide(x="Heave PPR", y="Heave Pitch") -> (x/y=→"Heave Pulses/mm":dbl)
        n3572 = Bundle By Name(cluster=w4758, "Heave and Surge COM Port:"=w4756) -> (w4757:T14)
        n3573 = Equal?(x=w4779, y=w4756) -> (x = y?=w4778:bool)
        n3574 = Divide(x="Sway PPR", y="Sway Pitch") -> (x/y=→"Sway Pulses/mm":dbl)
        n3575 = case shown="False" w4778 {
          tunnel: [w4783 w4800] -> w4777
          tunnel: w4759 -> [w4784 w4806]
          tunnel: w4757 -> [w4782 w4804]
          tunnel: [w4781 w4799] -> w4774
          frame False {
            n3576 = call <vilib>:"Clear Errors.vi"("error in (no error)"=w4784) -> ("error out"=w4780:errorcluster)  [unwired: 5 in, 1 out]
            n3577 = call "Instrument fgv.vi"("Enum"=T23."ERROR INIT", "error in (no error) 2"=w4780, "INPUT"=w4782) -> ("error"=w4786:errorcluster, "output"=w4781:T14)  [unwired: 6 in, 1 out]
            n3578 = call <vilib>:"Clear Errors.vi"("error in (no error)"=w4786) -> ("error out"=w4783:errorcluster)  [unwired: 5 in, 1 out]
          }
          frame True {
            n3579 = call "Instrument fgv.vi"("Enum"=T23."READ", "error in (no error) 2"=w4806, "INPUT"=w4804) -> ("error"=w4805:errorcluster, "output"=w4796:T14)  [unwired: 6 in, 1 out]
            n3580 = Bundle By Name(cluster=w4796, "String 36"="String") -> (w4795:T14)
            n3581 = case shown="True" "Write S" {
              selector: "Write S" -> [_ w4826]
              tunnel: w4805 -> [w4819 w4825]
              tunnel: [w4819 w4824] -> w4792
              tunnel: w4795 -> [w4818 w4821]
              tunnel: [w4818 w4820] -> w4791
              frame False {
              }
              frame True {
                n3582 = Not(x=w4826) -> (.not. x?=w4822:bool)
                n3583 = local write "Write S"(w4822) -> ()
                n3584 = call "Instrument fgv.vi"("Enum"=T23."MANUAL WRITE", "error in (no error) 2"=w4825, "INPUT"=w4821) -> ("error"=w4824:errorcluster, "output"=w4820:T14)  [unwired: 6 in, 1 out]
              }
            }
            n3585 = Array Size(array="WriteHumidity") -> (size(s)=w4789:i32)
            n3586 = Greater Than 0?(x=w4789) -> (x > 0?=w4787:bool)
            n3587 = call "Instrument fgv.vi"("Enum"=T23."WRITE", "error in (no error) 2"=w4792, "WriteCC1"="WriteHumidity", "INPUT"=w4791) -> ("error"=w4802:errorcluster, "WriteCC1 2"=w4790:string[], "output"=w4801:T14)  [unwired: 5 in]
            n3588 = case shown="True" w4787 {
              tunnel: w4790 -> [_ w4808]
              frame False {
              }
              frame True {
                n3589 = local write "WriteHumidity"(w4808) -> ()
              }
            }
            n3590 = case shown="Error" w4802 {
              selector: w4802 -> [w4809 w4812]
              tunnel: w4801 -> [w4810 w4817]
              tunnel: [w4810 w4816] -> w4799
              tunnel: [w4809 w4814] -> w4800
              frame No Error {
              }
              frame Error {
                n3591 = call <vilib>:"Clear Errors.vi"("error in (no error)"=w4812) -> ("error out"=w4811:errorcluster)  [unwired: 5 in, 1 out]
                n3592 = call "Instrument fgv.vi"("Enum"=T23."ERROR INIT", "error in (no error) 2"=w4811, "INPUT"=w4817) -> ("error"=w4815:errorcluster, "output"=w4816:T14)  [unwired: 6 in, 1 out]
                n3593 = call <vilib>:"Clear Errors.vi"("error in (no error)"=w4815) -> ("error out"=w4814:errorcluster)  [unwired: 5 in, 1 out]
              }
            }
            n3594 = Unbundle By Name(w4799) -> ("LastCom"=→"LastCom":string, "Read Heave and Surge"=→"Read Humidity":string)
          }
        }
        n3595 = Divide(x="Surge PPR", y="Surge Pitch") -> (x/y=→"Surge Pulses/mm":dbl)
        n3596 = Unbundle By Name(w4774) -> ("Heave COM Status 2"=w4776:bool, "Heave COM Status"=w4775:bool, "Error Heave"=w4772:errorcluster, "Bytes at Heave Port"=→"Bytes at Humidity Port":dbl)
        n3597 = Unbundle By Name(w4772) -> ("status"=→"Humidity Port":bool)
        n3598 = local write "Error Heave"(w4772) -> ()
        n3599 = Not(x=w4775) -> (.not. x?=w4760:bool)
        n3600 = Not(x=w4776) -> (.not. x?=w4761:bool)
        n3601 = local write "Heave COM Status 2"(w4761) -> ()
        n3602 = local write "Instrument Status"(w4760) -> ()
        n3603 = local read "Quit"() -> (w4753:bool)
        n3604 = Select(t=enum16{"init", "MAIN", "Panel Close"}."Panel Close", s=w4753, f=enum16{"init", "MAIN", "Panel Close"}."MAIN") -> (s? t:f=w4752:enum16{"init", "MAIN", "Panel Close"})
      }
      frame "Panel Close" {
      }
      frame Default {
      }
    }
  }
  n3605 = while {
    stop <- w4857 stop-if-true
    n3606 = local read "Read Humidity"() -> (w4838:string)
    n3607 = call <vilib>:"High Resolution Polling Wait.vi"("seconds to wait"=0.1) -> ()  [unwired: 10 in, 1 out]
    n3608 = Spreadsheet String To Array(delimiter (Tab)=",", format string="", spreadsheet string=w4838, array type (2D Dbl)=string[] []) -> (array=w4852:string[])
    n3609 = for {
      tunnel: w4852 -> [w4862] mode=indexing
      tunnel: string[] ["STATE;", "SET;", "RH;", "T;", "AMB_RH;", "AMB_T;", "PUMP;", "FAN_IN;", "FAN_OUT;", "DEHUM;", "CURRENT;", "STALL;"] -> [w4861] mode=indexing
      tunnel: [w4860] -> w4851 mode=indexing
      n3610 = Match Pattern(string=w4862, regular expression=w4861) -> (after substring=w4860:string)  [unwired: 1 in, 3 out]
    }
    n3611 = Index Array(array=w4851) -> (element #1=→"STATE :":string, element #2=→"SET :":string, element #3=w4840:string, element #4=→"T :":string, element #5=w4837:string, element #6=→"AMB_T :":string, element #7=→"PUMP :":string, element #8=→"FAN_IN :":string, element #9=→"FAN_OUT :":string, element #10=→"DEHUM :":string, element #11=→"CURRENT :":string, element #12=→"STALL :":string)  [unwired: 12 in]
    "RH :" <- w4840
    "AMB_RH :" <- w4837
    n3612 = Fract/Exp String To Number(string=w4840) -> (number=w4832:dbl)  [unwired: 3 in, 1 out]
    n3613 = Fract/Exp String To Number(string=w4837) -> (number=w4836:dbl)  [unwired: 3 in, 1 out]
    n3614 = local write "Ambient Humidity :"(w4836) -> ()
    n3615 = Equal?(x=w4832, y=0.0) -> (x = y?=w4834:bool)
    n3616 = case shown="True" w4834 {
      tunnel: [w4858 w4859] -> w4833
      tunnel: w4832 -> [w4858 _]
      frame False {
        (unwired) 0.0
        "Humidity temp" <- w4858
      }
      frame True {
        n3617 = local read "Humidity temp"() -> (w4859:dbl)
      }
    }
    "RH Numeric:" <- w4833
    n3618 = local read "Quit"() -> (w4857:bool)
  }
  n3619 = disable-structure shown="Disabled" {
    frame Disabled {
      n3620 = while {
        tunnel: [w5096] -> _
        i -> [w5096]
